vi "SVN_prepareCodebase.vi"(8 "error in (no error)":errorcluster, 10 "URL":string="https://svn.cim.as/svn/CIM_TM/Projects/3173 SVS - SmartVisionSystem/LV2016/trunk/LabVIEW", 11 "WorkingCopy":string="C:\\temp\\Workspace1") -> (0 "error out":errorcluster, 1 "standard error":string, 2 "standard output":string, 3 "WrokingCopy out":string="C:\\temp\\Workspace1")   [LabVIEW 2017]
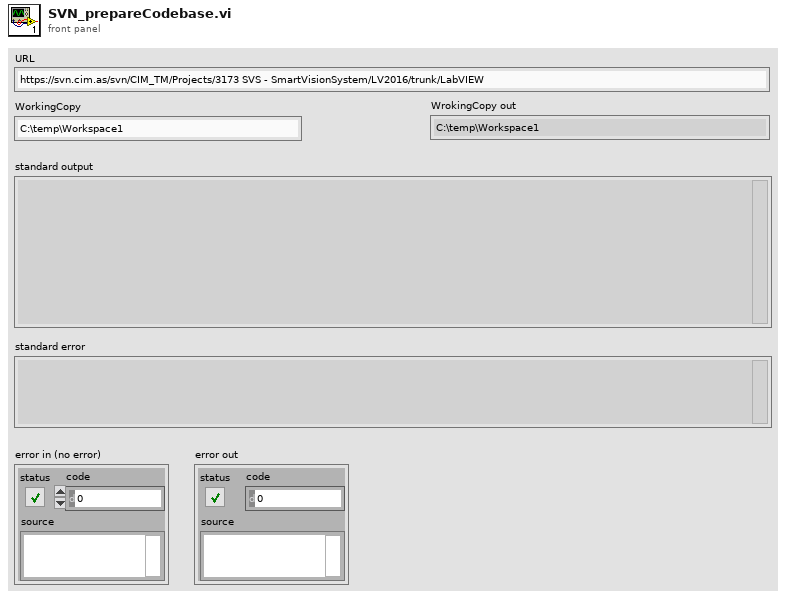
[diagram p1: front panel]
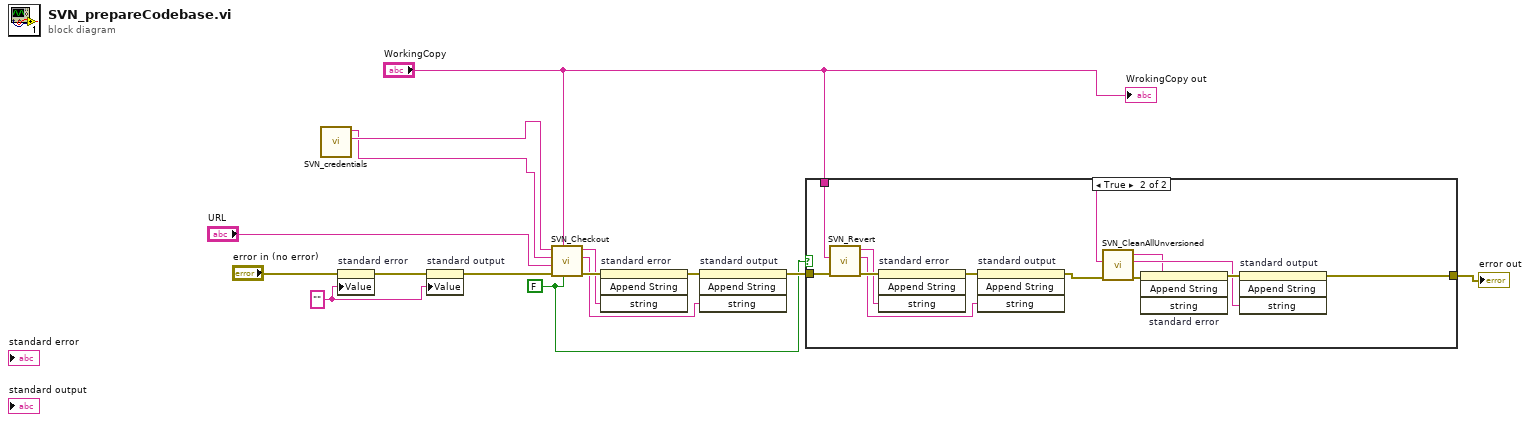
[diagram p0: block diagram]
diagram:
  w3 = FALSE ("checkout? (T)")
  w11 = "" ("standard error")
  n1 = call "SVN_credentials.vi"() -> ("Username"=w2:string, "Password"=w1:string)  [unwired: 10 in]
  n2 = property on="standard error" class="Str"(error in="error in (no error)", "Value"=w11) -> (error out=w13:errorcluster)  [unwired: 1 in, 1 out]
  n3 = property on="standard output" class="Str"(error in=w13, "Value"=w11) -> (error out=w12:errorcluster)  [unwired: 1 in, 1 out]
  n4 = call "SVN_Checkout.vi"("checkout? (T)"=w3, "Path"="WorkingCopy", "error in (no error)"=w12, "URL"="URL", "Password"=w1, "Username"=w2) -> ("error out"=w10:errorcluster, "standard output"=w8:string, "standard error"=w7:string)  [unwired: 2 in, 1 out]
  n5 = invoke on="standard error" class="Str" method="Append String"(error in=w10, "string"=w7) -> (error out=w9:errorcluster)  [unwired: 2 in, 3 out]
  n6 = invoke on="standard output" class="Str" method="Append String"(error in=w9, "string"=w8) -> (error out=w6:errorcluster)  [unwired: 2 in, 3 out]
  n7 = case shown="True" w3 {
    tunnel: w6 -> [w16 w26]
    tunnel: "WorkingCopy" -> [_ w18]
    tunnel: [w16 w17] -> w4
    frame False {
    }
    frame True {
      n8 = call "SVN_Revert.vi"("error in (no error)"=w26, "WorkingCopy"=w18) -> ("error out"=w28:errorcluster, "standard output"=w24:string, "standard error"=w27:string)  [unwired: 6 in, 1 out]
      n9 = invoke on="standard error" class="Str" method="Append String"(error in=w28, "string"=w27) -> (error out=w25:errorcluster)  [unwired: 2 in, 3 out]
      n10 = invoke on="standard output" class="Str" method="Append String"(error in=w25, "string"=w24) -> (error out=w23:errorcluster)  [unwired: 2 in, 3 out]
      n11 = call "SVN_CleanAllUnversioned.vi"("error in (no error)"=w23, "Path"=w18) -> ("error out"=w21:errorcluster, "standard output"=w20:string, "standard error"=w19:string)  [unwired: 6 in, 1 out]
      n12 = invoke on="standard error" class="Str" method="Append String"(error in=w21, "string"=w19) -> (error out=w22:errorcluster)  [unwired: 2 in, 3 out]
      n13 = invoke on="standard output" class="Str" method="Append String"(error in=w22, "string"=w20) -> (error out=w17:errorcluster)  [unwired: 2 in, 3 out]
    }
  }
  "error out" <- w4
  "WrokingCopy out" <- "WorkingCopy"
